vi "TDC_getSignalConditioning.vi"(5 "Channel":i32, 11 "Error In":errorcluster) -> (6 "Edge":i32(ring)=1 items=["Falling", "Rising"], 10 "threshold":dbl format="%#_6pV", 15 "Error Out":errorcluster)   [LabVIEW 2011]
uses:
  tdcbase.dll
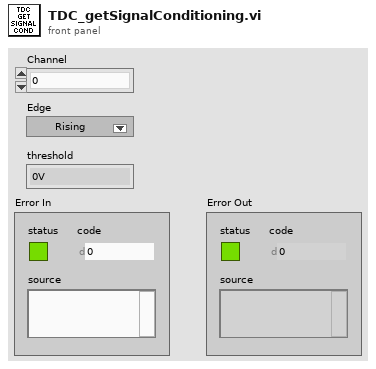
[diagram p1: front panel]
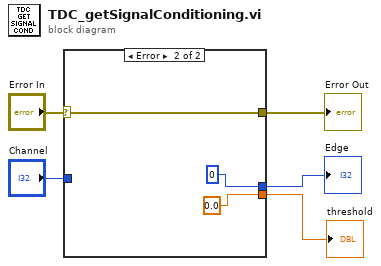
[diagram p0: block diagram]
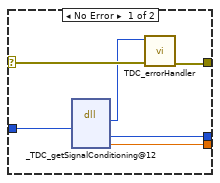
[diagram p2: hidden frame]
diagram:
  n1 = case shown="Error" "Error In" {
    selector: "Error In" -> [w11 w14]
    tunnel: [w10 w14] -> w4
    tunnel: "Channel" -> [w8 _]
    tunnel: [w7 0] -> w2
    tunnel: [w6 0.0] -> w1
    frame No Error {
      n2 = dll-call lib="X:/tdcbase.dll" fn="_TDC_getSignalConditioning@12"("channel"=w8) -> ("return type"=w9:i32, "edge"=w7:i32, "threshold"=w6:dbl)  [unwired: 6 in, 2 out]
      n3 = call "TDC_errorHandler.vi"("Error In"=w11, "TDC Return Code"=w9) -> ("Error Out"=w10:errorcluster)  [unwired: 9 in]
    }
    frame Error {
    }
  }
  "Error Out" <- w4
  "Edge" <- w2
  "threshold" <- w1
